vi "RichToFlatnixnet_grpc_WriteStateValue.vi"(5 "OutputClusterType":T1, 11 "InputCluster":T4) -> (3 "OutputCluster":T1)   [LabVIEW 2025, in "grpc-xnet_client.lvlib"]
uses:
  grpc-xnet_client.lvlib
  nixnet_grpc_WriteStateValue.ctl
  nixnet_grpc_WriteStateValue_value/nixnet_grpc_WriteStateValue_value.lvclass
  nixnet_grpc_WriteStateValue_Flat.ctl
  nixnet_grpc_LinDiagnosticScheduleChangeRequest_Flat.ctl
  nixnet_grpc_LinDiagnosticSchedule.ctl
  nixnet_grpc_WriteStateValue_value/nixnet_grpc_WriteStateValue_value.lvclass/nixnet_grpc_WriteStateValue_value.ctl
  nixnet_grpc_LinDiagnosticScheduleChangeRequest_schedule_enum/nixnet_grpc_LinDiagnosticScheduleChangeRequest_schedule_enum.lvclass/nixnet_grpc_LinDiagnosticScheduleChangeRequest_schedule_enum.ctl
  nixnet_grpc_LinDiagnosticScheduleChangeRequest_schedule_enum/Getschedule.vi
  nixnet_grpc_LinDiagnosticScheduleChangeRequest_schedule_enum/Getschedule_raw.vi
  nixnet_grpc_LinDiagnosticScheduleChangeRequest_schedule_enum/nixnet_grpc_LinDiagnosticScheduleChangeRequest_schedule_enum.lvclass
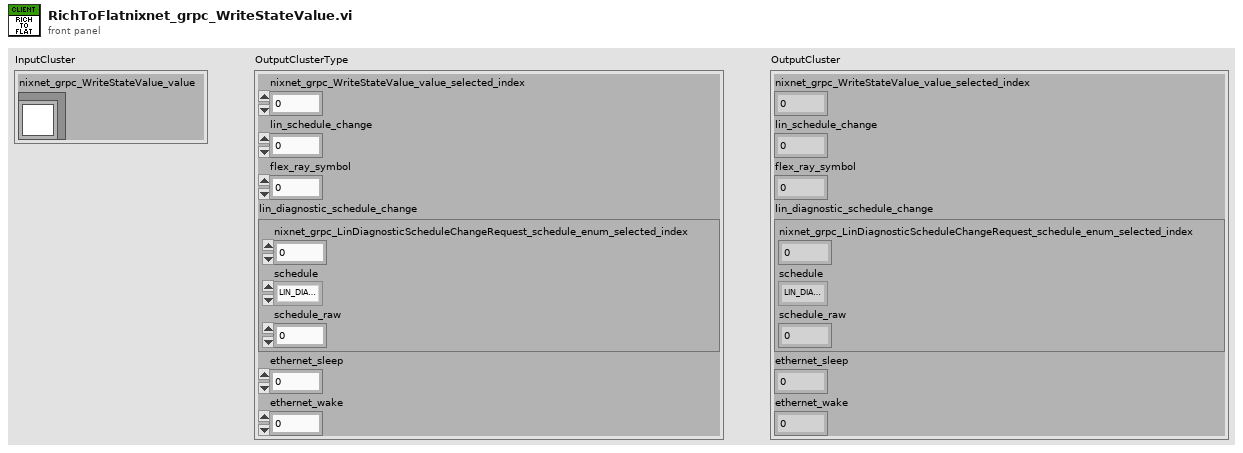
[diagram p1: front panel]
types:
  T1 = typedef "grpc-xnet_client.lvlib/nixnet_grpc_WriteStateValue_Flat.ctl" = cluster{"nixnet_grpc_WriteStateValue_value_selected_index":i32, "lin_schedule_change":u32, "flex_ray_symbol":u32, "lin_diagnostic_schedule_change":T2, "ethernet_sleep":u32, "ethernet_wake":u32}
  T2 = typedef "grpc-xnet_client.lvlib/nixnet_grpc_LinDiagnosticScheduleChangeRequest_Flat.ctl" = cluster{"nixnet_grpc_LinDiagnosticScheduleChangeRequest_schedule_enum_selected_index":i32, "schedule":T3, "schedule_raw":u32}
  T3 = typedef "grpc-xnet_client.lvlib/nixnet_grpc_LinDiagnosticSchedule.ctl" = enum32{"LIN_DIAGNOSTIC_SCHEDULE_NULL", "LIN_DIAGNOSTIC_SCHEDULE_MASTER_REQ", "LIN_DIAGNOSTIC_SCHEDULE_SLAVE_RESP"}
  T4 = typedef "grpc-xnet_client.lvlib/nixnet_grpc_WriteStateValue.ctl" = cluster{"nixnet_grpc_WriteStateValue_value":refnum<class "nixnet_grpc_WriteStateValue_value.lvclass">}
  T5 = typedef "grpc-xnet_client.lvlib/nixnet_grpc_LinDiagnosticScheduleChangeRequest.ctl" = cluster{"nixnet_grpc_LinDiagnosticScheduleChangeRequest_schedule_enum":refnum<class "nixnet_grpc_LinDiagnosticScheduleChangeRequest_schedule_enum.lvclass">}
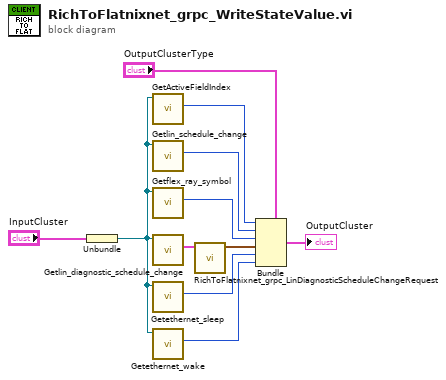
[diagram p0: block diagram]
diagram:
  n1 = Unbundle "Unbundle"("InputCluster") -> ("nixnet_grpc_WriteStateValue_value"=w8:refnum<class "nixnet_grpc_WriteStateValue_value.lvclass">)
  n2 = call "GetActiveFieldIndex.vi"("OneOfTemplate in"=w8) -> ("Active Field Index"=w7:i32)  [unwired: 8 in, 2 out]
  n3 = call "Getlin_schedule_change.vi"("OneOfTemplate in"=w8) -> ("Get_Val"=w6:u32)  [unwired: 8 in, 2 out]
  n4 = call "Getflex_ray_symbol.vi"("OneOfTemplate in"=w8) -> ("Get_Val"=w5:u32)  [unwired: 8 in, 2 out]
  n5 = call "Getlin_diagnostic_schedule_change.vi"("OneOfTemplate in"=w8) -> ("Get_Val"=w4:T5)  [unwired: 8 in, 2 out]
  n6 = call "Getethernet_sleep.vi"("OneOfTemplate in"=w8) -> ("Get_Val"=w2:u32)  [unwired: 8 in, 2 out]
  n7 = call "Getethernet_wake.vi"("OneOfTemplate in"=w8) -> ("Get_Val"=w1:u32)  [unwired: 8 in, 2 out]
  n8 = call "RichToFlatnixnet_grpc_LinDiagnosticScheduleChangeRequest.vi"("InputCluster"=w4) -> ("OutputCluster"=w3:T2)  [unwired: 10 in]
  n9 = Bundle "Bundle"(cluster="OutputClusterType", "nixnet_grpc_WriteStateValue_value_selected_index"=w7, "lin_schedule_change"=w6, "flex_ray_symbol"=w5, "lin_diagnostic_schedule_change"=w3, "ethernet_sleep"=w2, "ethernet_wake"=w1) -> (→"OutputCluster":T1)
